vi "USBTC08ChannelSetting.vi"(8 "error in (no error)":errorcluster, 10 "Channel Settings":T1 {"Type # 8" items=["B", "E", "J", "K", "N", "R", "S", "T", "Voltage"]; "Type # 7" items=["B", "E", "J", "K", "N", "R", "S", "T", "Voltage"]; "Type # 6" items=["B", "E", "J", "K", "N", "R", "S", "T", "Voltage"]; "Type # 5" items=["B", "E", "J", "K", "N", "R", "S", "T", "Voltage"]; "Type # 4" items=["B", "E", "J", "K", "N", "R", "S", "T", "Voltage"]; "Type # 3" items=["B", "E", "J", "K", "N", "R", "S", "T", "Voltage"]; "Type # 2" items=["B", "E", "J", "K", "N", "R", "S", "T", "Voltage"]; "Type # 1" items=["B", "E", "J", "K", "N", "R", "S", "T", "Voltage"]}, 11 "Handle In":i16) -> (0 "error out":errorcluster, 2 "Channel Enable Array":u8[](array[numeric]), 3 "Handle out":i16)   [LabVIEW 2009]
uses:
  usbtc08.dll
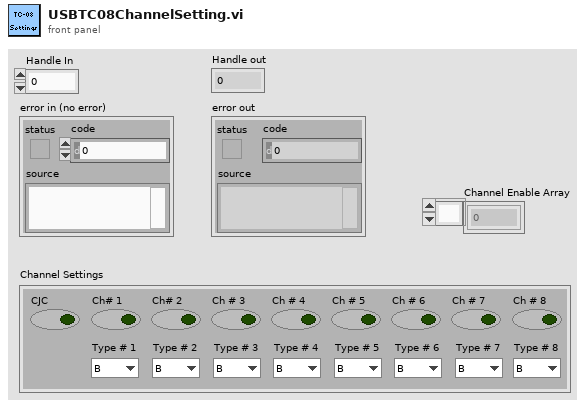
[diagram p1: front panel]
types:
  T1 = cluster{"Type # 1":i16, "Ch# 1":bool, "Type # 2":i16, "Ch# 2":bool, "Type # 3":i16, "Ch # 3":bool, "Type # 4":i16, "Ch # 4":bool, "Type # 5":i16, "Ch # 5":bool, "Type # 6":i16, "Ch # 6":bool, "Type # 7":i16, "Ch # 7":bool, "Type # 8":i16, "Ch # 8":bool, "CJC":bool}
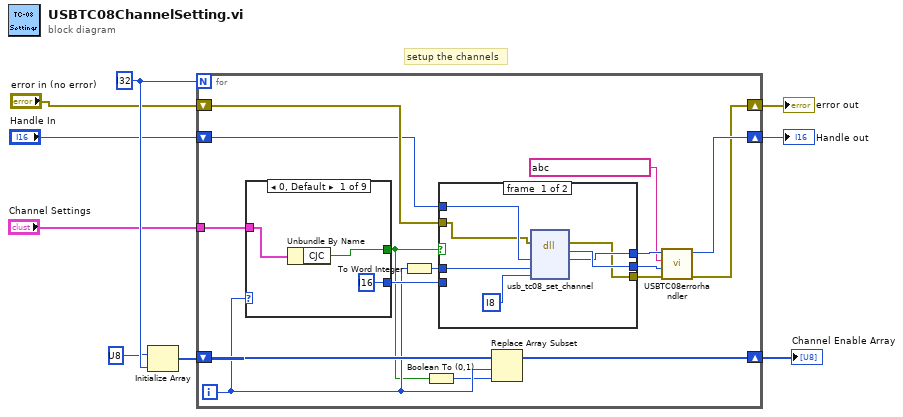
[diagram p0: block diagram]
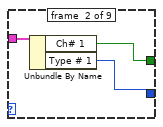
[diagram p2: hidden frame]
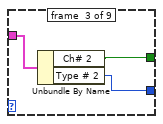
[diagram p3: hidden frame]
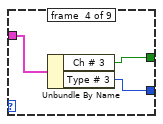
[diagram p4: hidden frame]
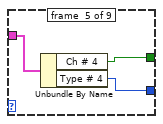
[diagram p5: hidden frame]
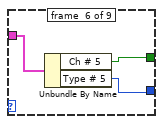
[diagram p6: hidden frame]
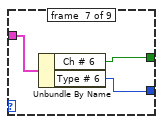
[diagram p7: hidden frame]
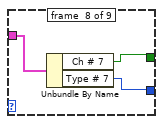
[diagram p8: hidden frame]
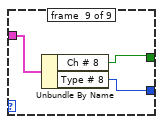
[diagram p9: hidden frame]
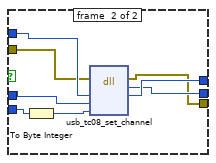
[diagram p10: hidden frame]
diagram:
  w7 = i32 ?
  # "setup the channels"
  n1 = Initialize Array(u8 ? ("element"), w7) -> (w5:u8[])
  n2 = for {
    N: w7 -> [_]
    shift-right: [w25] -> w8
    shift-left: w5 -> [w24]
    shift-right: [w17] -> w4
    shift-left: "Handle In" -> [w11]
    shift-right: [w13] -> w9
    shift-left: "error in (no error)" -> [w12]
    tunnel: "Channel Settings" -> [w10]
    i -> [w22]
    n3 = case shown="0, Default" w22 {
      tunnel: [w27 w30 w33 w36 w39 w42 w45 w48 w51] -> w21
      tunnel: [i16 ? ("Type # 2") w29 w32 w35 w38 w41 w44 w47 w50] -> w23
      tunnel: w10 -> [w26 w31 w34 w37 w40 w43 w46 w49 w52]
      frame #0 {
        n4 = Unbundle By Name(w26) -> ("CJC"=w27:bool)
      }
      frame #1 {
        n5 = Unbundle By Name(w31) -> ("Ch# 1"=w30:bool, "Type # 1"=w29:i16)
      }
      frame #2 {
        n6 = Unbundle By Name(w34) -> ("Ch# 2"=w33:bool, "Type # 2"=w32:i16)
      }
      frame #3 {
        n7 = Unbundle By Name(w37) -> ("Ch # 3"=w36:bool, "Type # 3"=w35:i16)
      }
      frame #4 {
        n8 = Unbundle By Name(w40) -> ("Ch # 4"=w39:bool, "Type # 4"=w38:i16)
      }
      frame #5 {
        n9 = Unbundle By Name(w43) -> ("Ch # 5"=w42:bool, "Type # 5"=w41:i16)
      }
      frame #6 {
        n10 = Unbundle By Name(w46) -> ("Ch # 6"=w45:bool, "Type # 6"=w44:i16)
      }
      frame #7 {
        n11 = Unbundle By Name(w49) -> ("Ch # 7"=w48:bool, "Type # 7"=w47:i16)
      }
      frame #8 {
        n12 = Unbundle By Name(w52) -> ("Ch # 8"=w51:bool, "Type # 8"=w50:i16)
      }
    }
    n13 = To Word Integer(number=w22) -> (16bit integer=w16:i16)
    n14 = Boolean To (0,1)(Boolean=w21) -> (0, 1=w20:i16)
    n15 = case shown="True" w21 {
      tunnel: w23 -> [_ w63]
      tunnel: [w57 w67] -> w19
      tunnel: [w58 w66] -> w18
      tunnel: w11 -> [w56 w65]
      tunnel: w16 -> [w55 w62]
      tunnel: w12 -> [w54 w61]
      tunnel: [w53 w60] -> w14
      frame #0 {
        n16 = dll-call lib="usbtc08.dll" fn="usb_tc08_set_channel"(error in=w54, "handle"=w56, "channel"=w55, "tc_type"=i8 ?) -> (error out=w53:errorcluster, "return type"=w58:i16, "handle"=w57:i16)  [unwired: 4 in, 1 out]
      }
      frame #1 {
        n17 = To Byte Integer(number=w63) -> (8bit integer=w64:i8)
        n18 = dll-call lib="usbtc08.dll" fn="usb_tc08_set_channel"(error in=w61, "handle"=w65, "channel"=w62, "tc_type"=w64) -> (error out=w60:errorcluster, "return type"=w66:i16, "handle"=w67:i16)  [unwired: 4 in, 1 out]
      }
    }
    n19 = Replace Array Subset(array=w24, new element=w20, index=w22) -> (w25:u8[])
    n20 = call "USBTC08errorhandler.vi"("error in (no error)"=w14, "Return"=w18, "API function"=string ?, "Handle in"=w19) -> ("error out"=w13:errorcluster, "Handle out"=w17:i16)  [unwired: 6 in]
  }
  "error out" <- w9
  "Channel Enable Array" <- w8
  "Handle out" <- w4
